vi "Event Loop Wrapper.vi"(8 "Error Q":refnum<queue>, 9 "Helper Loop Q":refnum<queue>, 10 "Actor":refnum<class "Actor.lvclass">, 11 "Helper Loop in":refnum<class "Helper Loop.lvclass">) -> ()   [LabVIEW 2021, in "Helper Loop.lvclass"]
uses:
  Helper Loop.lvclass
  <vilib>/jettl/jettl/Actor/Actor/Actor.lvclass
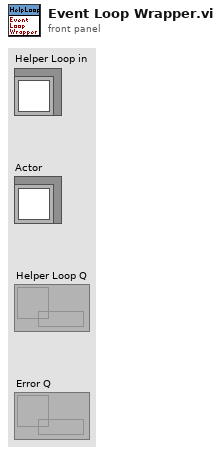
[diagram p1: front panel]
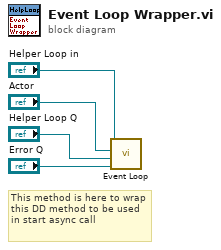
[diagram p0: block diagram]
diagram:
  # "This method is here to wrap this DD method to be used in start async call"
  n1 = call-dynamic "Event Loop.vi"("Error Q"="Error Q", "Helper Loop Q"="Helper Loop Q", "Actor"="Actor", "Helper Loop in"="Helper Loop in") -> ()  [unwired: 8 in]
